vi "XYZ Control.vi"(1 "Wave Queue":refnum<queue>, 2 "Camera Queue":refnum<queue>, 3 "XYZ Controller":refnum<queue>) -> (0 "error out":errorcluster)   [LabVIEW 2016]
uses:
  controls/CameraControlTypeDef.ctl
  controls/Microscope Settings.ctl
  controls/ColourCalibration.ctl
  controls/ModeEnum.ctl
  controls/xy.ctl
  <vilib>/DAQmx/read.llb/DAQmx Read (Analog DBL 1Chan 1Samp).vi
  <vilib>/DAQmx/create/channels.llb/DAQmx Create Channel (AI-Voltage-Basic).vi
  <vilib>/DAQmx/miscellaneous.llb/DAQmx Fill In Error Info.vi
panel:
  in  "stop 2":bool
  in  "Z Position":dbl(slide) scale=-20000.0..20000.0 scale format="%#_6p"
  out "Z Position Read":dbl
  in  "End":dbl
  in  "Start":dbl
  in  "Step":dbl
  in  "Z Stack":bool
  in  "Delay /ms":dbl=100.0
  in  "Go to Current":bool
  in  "Clear List":bool
  in  "Add Current Position Highlighted":bool
  in  "Add Current Position":bool
  in  "Save Images":bool
  in  "Cycle Positions":bool
  in  "Coordinate List":i32(listbox)
  in  "Previous":bool
  in  "Next":bool
  out "Filter":i16
  out "Y Position Read":dbl
  out "X Position Read":dbl
  in  "Filter":dbl
  in  "Y Position":dbl(slide) scale=-20000.0..20000.0 scale format="%#_6p"
  in  "X Position":dbl(slide) scale=-20000.0..20000.0 scale format="%#_4p"
  in  "stop":bool
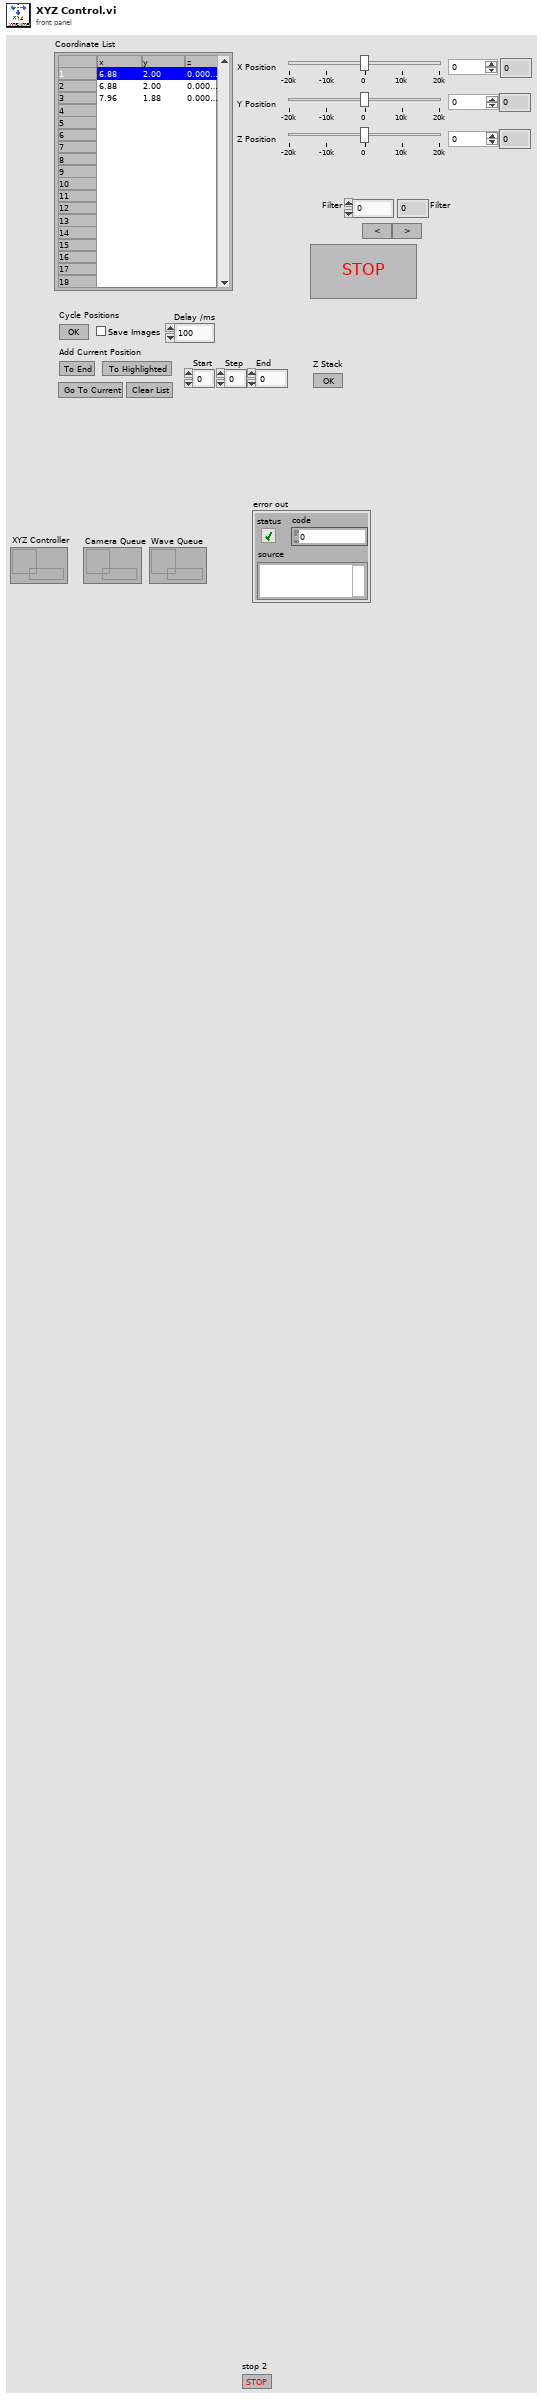
[diagram p1: front panel]
types:
  T1 = typedef "xy.ctl" = enum16{"Initalise", "setX", "getX", "setY", "getY", "stop", "setFilter", "getFilter", "FilterPrevious", "FilterNext", "setXYZ"}
  T2 = cluster{"State\n":T1, "X Position":dbl, "Y Position":dbl, "Filter":dbl, "Z Position":dbl}
  T3 = cluster{"Enum":T1, "X Position":dbl, "Y Position":dbl, "Filter":dbl, "Z Position":dbl}
  T4 = cluster{"State\n":T1, "X Position":dbl, "Y Position":dbl, dbl, "Filter":dbl}
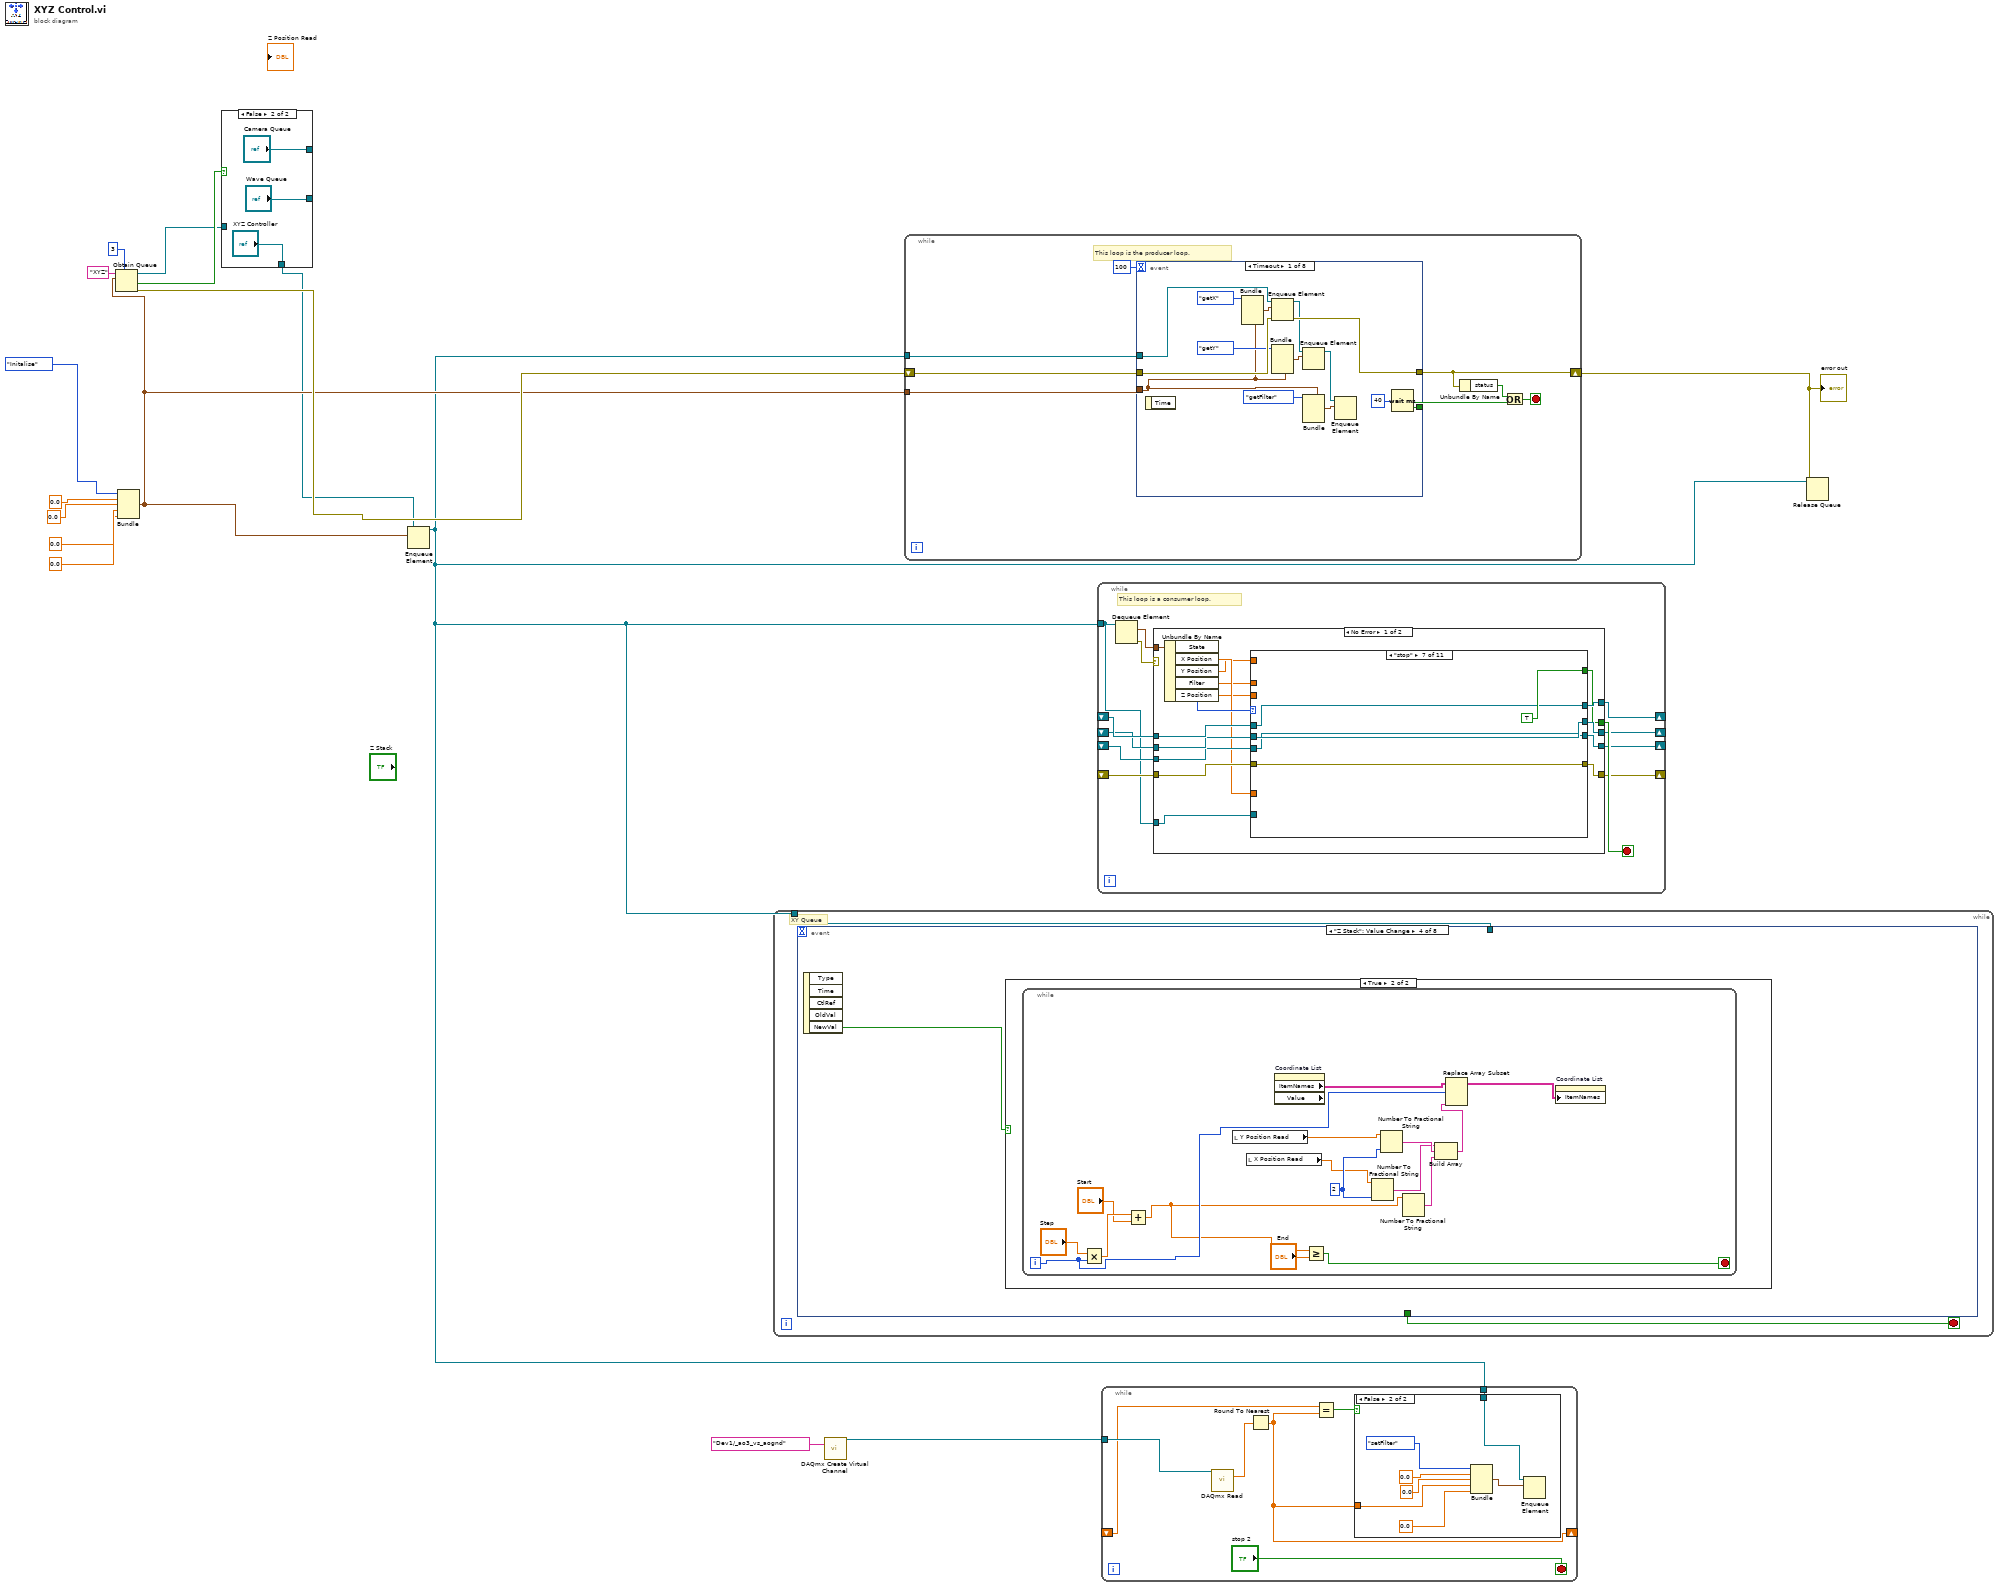
[diagram p0: block diagram]
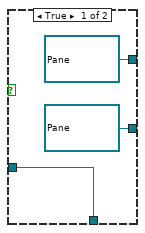
[diagram p3: hidden frame]
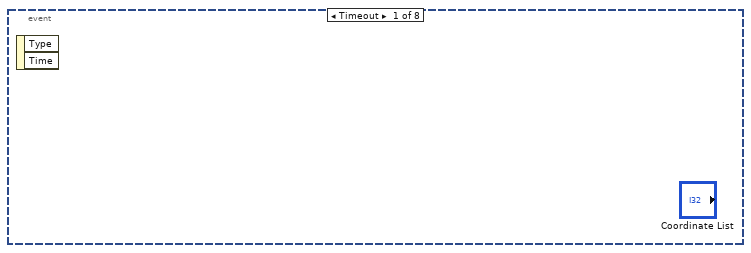
[diagram p4: hidden frame]
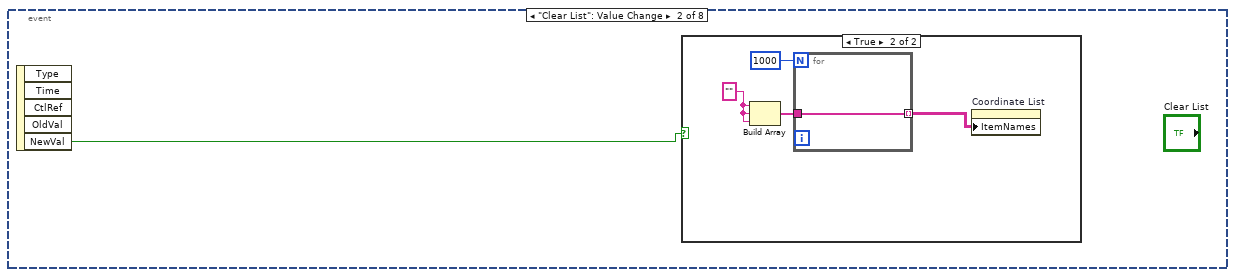
[diagram p5: hidden frame]
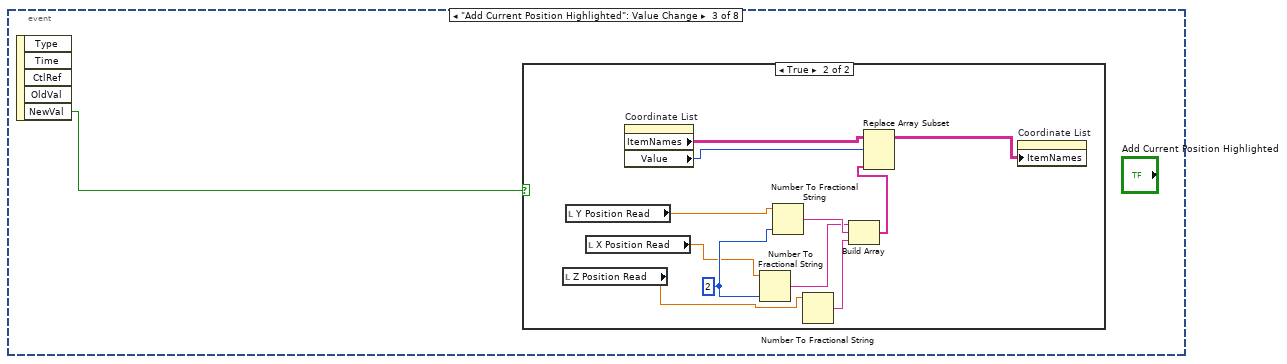
[diagram p7: hidden frame]
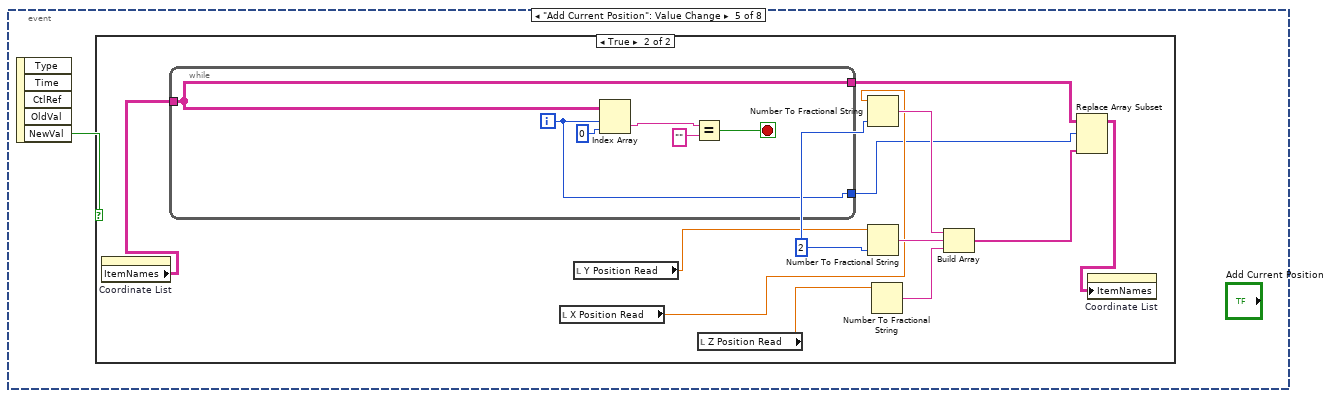
[diagram p10: hidden frame]
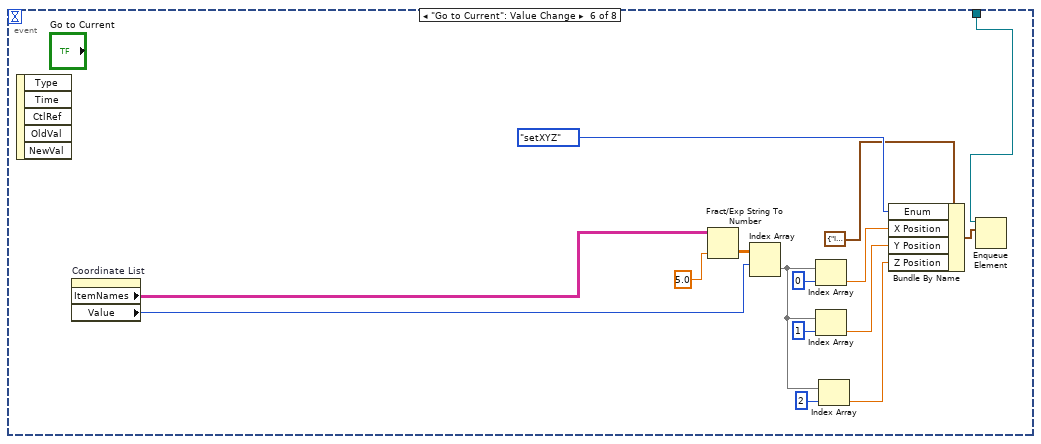
[diagram p12: hidden frame]
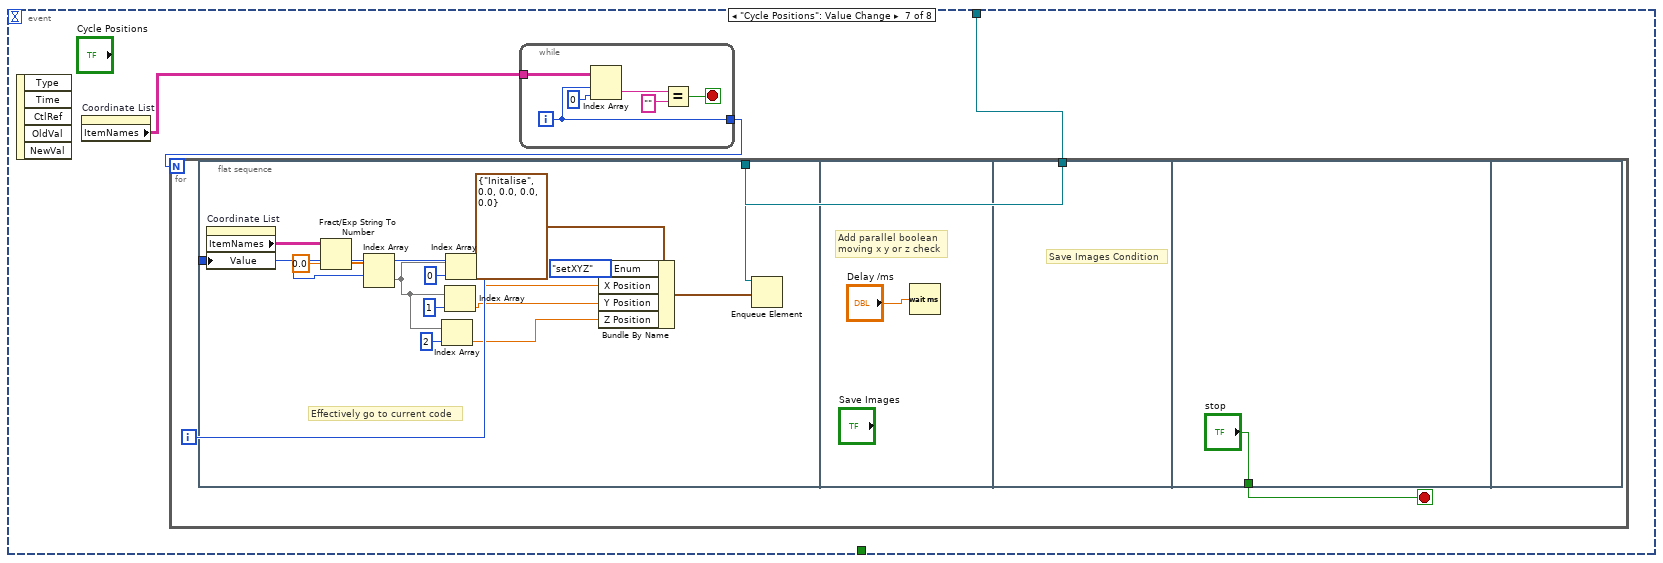
[diagram p13: hidden frame]
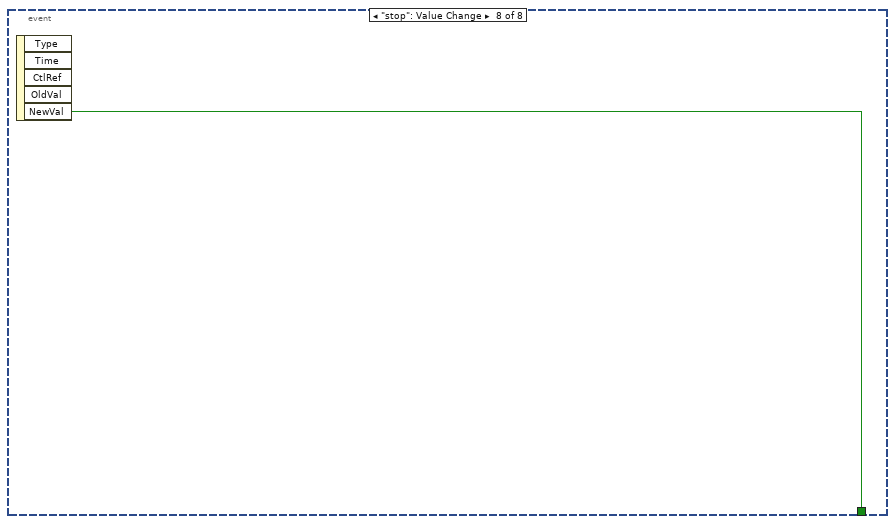
[diagram p14: hidden frame]
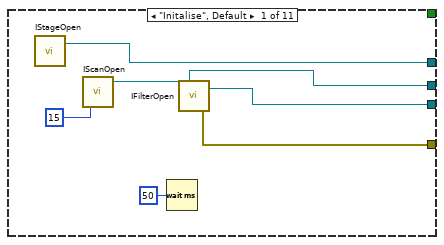
[diagram p15: hidden frame]
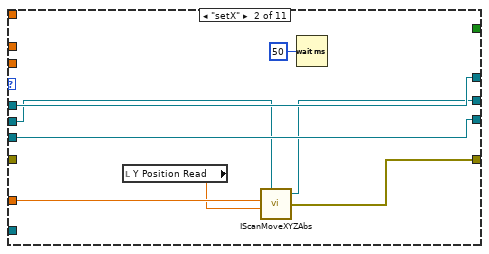
[diagram p16: hidden frame]
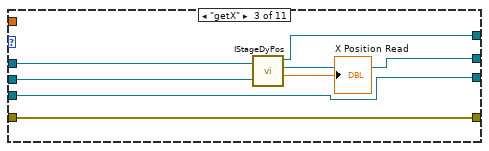
[diagram p17: hidden frame]
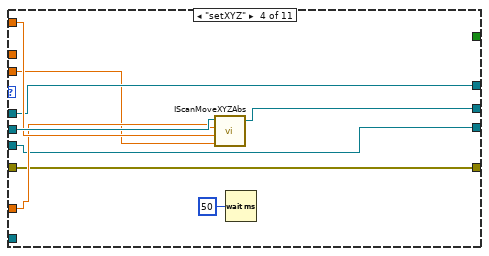
[diagram p18: hidden frame]
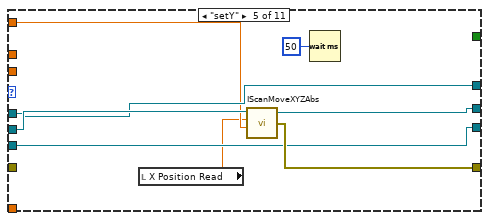
[diagram p19: hidden frame]
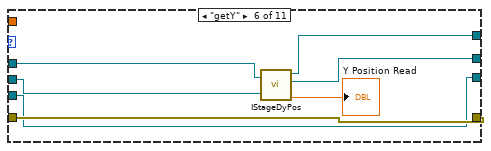
[diagram p20: hidden frame]
diagram:
  n1 = Bundle("State"=xy."Initalise", "X Position"=0.0, "Y Position"=0.0, "Filter"=0.0, "Z Position"=0.0) -> (w9:T2)  [unwired: 1 in]
  n2 = Obtain Queue(max queue size (-1, unlimited)=3, name (unnamed)="XYZ", element data type=w9) -> (queue out=w5:refnum<queue>, created new?=w6:bool, error out=w14:errorcluster)  [unwired: 2 in]
  n3 = case shown="False" w6 {
    tunnel: w5 -> [w19 _]
    tunnel: [w19 "XYZ Controller"] -> w4
    tunnel: [refnum<queue> refnum ("Wave Queue") "Wave Queue"] -> _
    tunnel: [refnum<queue> refnum ("Camera Queue") "Camera Queue"] -> _
    frame True {
    }
    frame False {
    }
  }
  n4 = Enqueue Element(queue=w4, element=w9) -> (queue out=w1:refnum<queue>)  [unwired: 2 in, 2 out]
  n5 = while {
    tunnel: w1 -> [w23]
    stop <- w24 stop-if-true
    # "XY Queue"
    n6 = event shown="[3] \"Z Stack\": Value Change" {
      selector: _ -> [_ _ _ _ _ _ _ _]
      dyn-events: _ -> [_ _ _ _ _ _ _ _]
      timeout: _ -> [_ _ _ _ _ _ _ _]
      tunnel: [_ _ _ _ _ _ _ w123] -> w24
      tunnel: w23 -> [_ _ _ _ _ w89 w94 _]
      event Timeout {
        n7 = event-data() -> ()  [unwired: 1 in, 2 out]
      }
      event "Clear List": Value Change {
        n8 = event-data() -> ("NewVal"=w25:bool)  [unwired: 1 in, 4 out]
        n9 = case shown="True" w25 {
          frame False {
          }
          frame True {
            w29 = "" ("y")
            n10 = Build Array(w29, w29, w29) -> (w27:string[])
            n11 = for {
              N: 1000 -> [_]
              tunnel: w27 -> [w30]
              tunnel: [w30] -> w26 mode=indexing
            }
            n12 = property on="Coordinate List" class="MCListbox (strict)"("ItemNames"=w26) -> ()  [unwired: 2 in, 2 out]
          }
        }
      }
      event "Add Current Position Highlighted": Value Change {
        n13 = event-data() -> ("NewVal"=w31:bool)  [unwired: 1 in, 4 out]
        n14 = case shown="True" w31 {
          frame False {
          }
          frame True {
            w39 = i16 2 ("width (-)")
            n15 = local read "Z Position Read"() -> (w32:dbl)
            n16 = local read "Y Position Read"() -> (w40:dbl)
            n17 = local read "X Position Read"() -> (w38:dbl)
            n18 = property on="Coordinate List" class="MCListbox (strict)"() -> ("ItemNames"=w41:string[][], "Value"=w42:i32)  [unwired: 2 in, 2 out]
            n19 = Number To Fractional String(number=w38, precision (6)=w39) -> (F-format string=w35:string)  [unwired: 2 in]
            n20 = Number To Fractional String(number=w40, precision (6)=w39) -> (F-format string=w36:string)  [unwired: 2 in]
            n21 = Number To Fractional String(number=w32) -> (F-format string=w37:string)  [unwired: 3 in]
            n22 = Build Array(w35, w36, w37) -> (w34:string[])
            n23 = Replace Array Subset(array=w41, new element=w34, index (row)=w42) -> (w33:string[][])  [unwired: 1 in]
            n24 = property on="Coordinate List" class="MCListbox (strict)"("ItemNames"=w33) -> ()  [unwired: 2 in, 2 out]
          }
        }
      }
      event "Z Stack": Value Change {
        n25 = event-data() -> ("NewVal"=w43:bool)  [unwired: 1 in, 4 out]
        n26 = case shown="True" w43 {
          frame False {
          }
          frame True {
            n27 = while {
              i -> [w58]
              stop <- w53 stop-if-true
              w50 = i16 2 ("width (-)")
              n28 = Multiply(x="Step", y=w58) -> (x*y=w57:dbl)
              n29 = Add(x=w57, y="Start") -> (x+y=w55:dbl)
              n30 = local read "Y Position Read"() -> (w51:dbl)
              n31 = local read "X Position Read"() -> (w49:dbl)
              n32 = property on="Coordinate List" class="MCListbox (strict)" props=["ItemNames", "Value"]() -> ("ItemNames"=w52:string[][])  [unwired: 2 in, 3 out]
              n33 = Greater Or Equal?(x=w55, y="End") -> (x >= y?=w53:bool)
              n34 = Number To Fractional String(number=w49, precision (6)=w50) -> (F-format string=w46:string)  [unwired: 2 in]
              n35 = Number To Fractional String(number=w51, precision (6)=w50) -> (F-format string=w47:string)  [unwired: 2 in]
              n36 = Number To Fractional String(number=w55) -> (F-format string=w48:string)  [unwired: 3 in]
              n37 = Build Array(w46, w47, w48) -> (w45:string[])
              n38 = Replace Array Subset(array=w52, new element=w45, index (row)=w58) -> (w44:string[][])  [unwired: 1 in]
              n39 = property on="Coordinate List" class="MCListbox (strict)"("ItemNames"=w44) -> ()  [unwired: 2 in, 2 out]
            }
          }
        }
      }
      event "Add Current Position": Value Change {
        n40 = event-data() -> ("NewVal"=w60:bool)  [unwired: 1 in, 4 out]
        n41 = case shown="True" w60 {
          frame False {
          }
          frame True {
            w69 = i16 2 ("precision (6)")
            n42 = property on="Coordinate List" class="MCListbox (strict)"() -> ("ItemNames"=w66:string[][])  [unwired: 2 in, 2 out]
            n43 = while {
              tunnel: [w75] -> w63
              tunnel: w66 -> [w74]
              tunnel: [w74] -> w65
              i -> [w75]
              stop <- w76 stop-if-true
              n44 = Index Array(array=w74, index (row)=w75, index (col)=0 ("disabled index (col)")) -> (element=w73:string)
              n45 = Equal?(x=w73, y="") -> (x = y?=w76:bool)
            }
            n46 = local read "X Position Read"() -> (w68:dbl)
            n47 = local read "Y Position Read"() -> (w67:dbl)
            n48 = local read "Z Position Read"() -> (w61:dbl)
            n49 = Number To Fractional String(number=w68, precision (6)=w69) -> (F-format string=w72:string)  [unwired: 2 in]
            n50 = Number To Fractional String(number=w67, precision (6)=w69) -> (F-format string=w70:string)  [unwired: 2 in]
            n51 = Number To Fractional String(number=w61) -> (F-format string=w71:string)  [unwired: 3 in]
            n52 = Build Array(w72, w70, w71) -> (w64:string[])
            n53 = Replace Array Subset(array=w65, new element=w64, index (row)=w63) -> (w62:string[][])  [unwired: 1 in]
            n54 = property on="Coordinate List" class="MCListbox (strict)"("ItemNames"=w62) -> ()  [unwired: 2 in, 2 out]
          }
        }
      }
      event "Go to Current": Value Change {
        n55 = event-data() -> ()  [unwired: 1 in, 5 out]
        n56 = property on="Coordinate List" class="MCListbox (strict)"() -> ("ItemNames"=w93:string[][], "Value"=w82:i32)  [unwired: 2 in, 2 out]
        n57 = Fract/Exp String To Number(string=w93, default (0 dbl)=5.0 ("default (0 DBL)")) -> (number=w92:dbl[][])  [unwired: 2 in, 1 out]
        n58 = Index Array(array=w92, index (row)=w82) -> (element=w80:dbl[])  [unwired: 1 in]
        n59 = Index Array(array=w80, index=0) -> (element=w84:dbl)
        n60 = Index Array(array=w80, index=1) -> (element=w85:dbl)
        n61 = Index Array(array=w80, index=2) -> (element=w79:dbl)
        n62 = Bundle By Name(cluster=T3 {"Enum"=enum."Initalise", "X Position"=0.0, "Y Position"=0.0, "Filter"=0.0, "Z Position"=0.0} ("element"), "Enum"=xy."setXYZ", "X Position"=w84, "Y Position"=w85, "Z Position"=w79) -> (w86:T3)
        n63 = Enqueue Element(queue=w89, element=w86) -> ()  [unwired: 2 in, 3 out]
      }
      event "Cycle Positions": Value Change {
        n64 = event-data() -> ()  [unwired: 1 in, 5 out]
        n65 = property on="Coordinate List" class="MCListbox (strict)"() -> ("ItemNames"=w96:string[][])  [unwired: 2 in, 2 out]
        n66 = while {
          tunnel: w96 -> [w122]
          tunnel: [w117] -> w95
          i -> [w117]
          stop <- w118 stop-if-true
          n67 = Index Array(array=w122, index (row)=w117, index (col)=0 ("disabled index (col)")) -> (element=w120:string)
          n68 = Equal?(x=w120, y="") -> (x = y?=w118:bool)
        }
        n69 = for {
          N: w95 -> [_]
          tunnel: w94 -> [w99]
          i -> [w98]
          stop <- w97 stop-if-true
          n70 = flat-sequence {
            tunnel: w99 -> [w103]
            tunnel: w98 -> [w101]
            tunnel: ["stop"] -> w97
            frame #0 {
              # "Effectively go to current code"
              n71 = property on="Coordinate List" class="MCListbox (strict)"("Value"=w101) -> ("ItemNames"=w102:string[][])  [unwired: 2 in, 2 out]
              n72 = Fract/Exp String To Number(string=w102, default (0 dbl)=0.0 ("default (0 DBL)")) -> (number=w114:dbl[][])  [unwired: 2 in, 1 out]
              n73 = Index Array(array=w114, index (row)=w101) -> (element=w112:dbl[])  [unwired: 1 in]
              n74 = Index Array(array=w112, index=2) -> (element=w100:dbl)
              n75 = Index Array(array=w112, index=1) -> (element=w106:dbl)
              n76 = Index Array(array=w112, index=0) -> (element=w107:dbl)
              n77 = Bundle By Name(cluster=T3 {"Enum"=enum."Initalise", "X Position"=0.0, "Y Position"=0.0, "Filter"=0.0, "Z Position"=0.0} ("element"), "Enum"=xy."setXYZ", "X Position"=w107, "Y Position"=w106, "Z Position"=w100) -> (w104:T3)
              n78 = Enqueue Element(queue=w103, element=w104) -> ()  [unwired: 2 in, 3 out]
            }
            frame #1 {
              # "Add parallel boolean\nmoving x y or z check"
              n79 = Wait (ms)(milliseconds to wait="Delay /ms") -> ()  [unwired: 1 out]
            }
            frame #2 {
              # "Save Images Condition"
            }
            frame #3 {
            }
            frame #4 {
            }
          }
        }
      }
      event "stop": Value Change {
        n80 = event-data() -> ("NewVal"=w123:bool)  [unwired: 1 in, 4 out]
      }
    }
  }
  n81 = call-poly <vilib>:"DAQmx Create Virtual Channel.vi"("physical channels"=tag "Dev1/_ao3_vs_aognd") -> ("task out"=w3:refnum<k21>)  [unwired: 13 in, 1 out]
  n82 = while {
    shift-right: [w127] -> w16
    shift-left: w14 -> [w130]
    tunnel: w1 -> [w131]
    tunnel: w9 -> [w125]
    stop <- w128 stop-if-true
    # "This loop is the producer loop."
    n83 = event shown="[0] Timeout" {
      selector: _ -> [_ _ _ _ _ _ _ _]
      dyn-events: _ -> [_ _ _ _ _ _ _ _]
      timeout: 100 -> [_ _ _ _ _ _ _ _]
      tunnel: w131 -> [w144 w148 w154 w163 w170 w173 w180 w191]
      tunnel: w130 -> [w143 w145 w153 w159 w169 _ _ w190]
      tunnel: [w140 _ _ w158 w167 _ _ w187] -> w127
      tunnel: [_ _ _ TRUE ("stop") _ _ _ _] -> w129
      tunnel: w125 -> [w139 w146 w152 w162 w168 w172 w179 w189]
      event Timeout {
        n84 = event-data() -> ()  [unwired: 1 in, 1 out]
        n85 = Bundle(cluster=w139, "State"=xy."getX") -> (w136:T2)  [unwired: 4 in]
        n86 = Enqueue Element(queue=w144, element=w136, error in (no error)=w143) -> (queue out=w137:refnum<queue>, error out=w140:errorcluster)  [unwired: 1 in, 1 out]
        n87 = Bundle(cluster=w139, "State"=xy."getY") -> (w135:T2)  [unwired: 4 in]
        n88 = Enqueue Element(queue=w137, element=w135) -> (queue out=w134:refnum<queue>)  [unwired: 2 in, 2 out]
        n89 = Bundle(cluster=w139, "State"=xy."getFilter") -> (w133:T2)  [unwired: 4 in]
        n90 = Enqueue Element(queue=w134, element=w133) -> ()  [unwired: 2 in, 3 out]
        n91 = Wait (ms)(milliseconds to wait=u32 40) -> ()  [unwired: 1 out]
      }
      event "Z Position": Value Change {
        n92 = event-data() -> ()  [unwired: 1 in, 2 out]
        n93 = Bundle(cluster=w146, "State"=xy."setX", "X Position"="Z Position") -> (w149:T2)  [unwired: 3 in]
        n94 = Enqueue Element(queue=w148, element=w149, error in (no error)=w145) -> ()  [unwired: 1 in, 3 out]
      }
      event "X Position": Value Change {
        n95 = event-data() -> ()  [unwired: 1 in, 1 out]
        n96 = Bundle(cluster=w152, "State"=xy."setX", "X Position"="X Position") -> (w155:T2)  [unwired: 3 in]
        n97 = Enqueue Element(queue=w154, element=w155, error in (no error)=w153) -> ()  [unwired: 1 in, 3 out]
      }
      event "stop": Value Change {
        n98 = event-data() -> ()  [unwired: 1 in, 1 out]
        n99 = Bundle(cluster=w162, "State"=xy."stop") -> (w160:T2)  [unwired: 4 in]
        n100 = Enqueue Element At Opposite End(queue=w163, element=w160, error in (no error)=w159) -> (error out=w158:errorcluster)  [unwired: 1 in, 2 out]
      }
      event "Filter": Value Change {
        n101 = event-data() -> ()  [unwired: 1 in, 1 out]
        n102 = Bundle(cluster=w168, "State"=xy."setFilter", "Filter"="Filter") -> (w166:T2)  [unwired: 3 in]
        n103 = Enqueue Element(queue=w170, element=w166, error in (no error)=w169) -> (error out=w167:errorcluster)  [unwired: 1 in, 2 out]
      }
      event "Next": Value Change {
        n104 = event-data() -> ()  [unwired: 1 in, 1 out]
        n105 = case shown="True" "Next" {
          tunnel: w173 -> [_ w176]
          tunnel: w172 -> [_ w175]
          frame False {
          }
          frame True {
            n106 = Bundle(cluster=w175, "State"=xy."FilterNext") -> (w174:T2)  [unwired: 4 in]
            n107 = Enqueue Element(queue=w176, element=w174) -> ()  [unwired: 2 in, 3 out]
          }
        }
      }
      event "Previous": Value Change {
        n108 = event-data() -> ()  [unwired: 1 in, 1 out]
        n109 = case shown="True" "Previous" {
          tunnel: w180 -> [_ w183]
          tunnel: w179 -> [_ w182]
          frame False {
          }
          frame True {
            n110 = Bundle(cluster=w182, "State"=xy."FilterPrevious") -> (w181:T2)  [unwired: 4 in]
            n111 = Enqueue Element(queue=w183, element=w181) -> ()  [unwired: 2 in, 3 out]
          }
        }
      }
      event "Y Position": Value Change {
        n112 = event-data() -> ()  [unwired: 1 in, 1 out]
        n113 = Bundle(cluster=w189, "State"=xy."setY", "Y Position"="Y Position") -> (w188:T2)  [unwired: 3 in]
        n114 = Enqueue Element(queue=w191, element=w188, error in (no error)=w190) -> (error out=w187:errorcluster)  [unwired: 1 in, 2 out]
      }
    }
    n115 = Unbundle By Name(w127) -> ("status"=w126:bool)
    n116 = Or(x=w126, y=w129) -> (x .or. y?=w128:bool)
  }
  "error out" <- w16
  n117 = while {
    tunnel: w1 -> [w192]
    shift-right: [w200] -> _
    shift-left: _ -> [w197]
    shift-right: [w199] -> _
    shift-left: _ -> [w196]
    shift-right: [w198] -> _
    shift-left: _ -> [w195]
    shift-right: [w194] -> _
    shift-left: _ -> [w193]
    stop <- w201 stop-if-true
    # "This loop is a consumer loop."
    n118 = Dequeue Element(queue=w192) -> (element=w202:T2, error out=w203:errorcluster)  [unwired: 2 in, 2 out]
    n119 = case shown="No Error" w203 {
      tunnel: w202 -> [w219 _]
      tunnel: [w209 TRUE] -> w201
      tunnel: [w217 _] -> w200
      tunnel: [w216 _] -> w199
      tunnel: [w215 _] -> w198
      tunnel: w197 -> [w214 _]
      tunnel: w196 -> [w213 _]
      tunnel: w195 -> [w212 _]
      tunnel: [w211 w294] -> w194
      tunnel: w193 -> [w210 w294]
      tunnel: w192 -> [w206 _]
      frame No Error {
        n120 = Unbundle By Name(w219) -> ("State"=w218:T1, "X Position"=w208:dbl, "Y Position"=w207:dbl, "Filter"=w204:dbl, "Z Position"=w205:dbl)
        n121 = case shown="\"stop\"" w218 {
          tunnel: [w225 w233 w238 w245 w254 w262 w267 w271 w277 w286 w289] -> w217
          tunnel: [w224 w229 w237 w246 w256 w261 w266 w272 w278 w287 w288] -> w216
          tunnel: [w223 w232 w235 w244 w253 w259 w265 w275 w279 w283 w292] -> w215
          tunnel: w214 -> [_ w233 w240 w245 w254 w264 w267 w271 w277 w286 w289]
          tunnel: w213 -> [_ w230 w239 w249 w257 w263 w266 w272 w278 w287 w288]
          tunnel: w212 -> [_ w232 w235 w244 w253 w259 w265 w274 w280 w284 w293]
          tunnel: [w222 w228 w236 w243 w255 w260 w269 w270 w281 w282 w291] -> w211
          tunnel: w210 -> [_ _ w236 w243 _ w260 w269 _ _ _ _]
          tunnel: [_ _ _ _ _ _ TRUE _ _ _ _] -> w209
          tunnel: w208 -> [_ w231 _ w247 _ _ _ _ _ _ _]
          tunnel: w207 -> [_ _ _ w248 w252 _ _ _ _ _ _]
          tunnel: w206 -> [_ _ _ _ _ _ _ _ _ _ _]
          tunnel: w205 -> [_ _ _ w241 _ _ _ _ _ _ _]
          tunnel: w204 -> [_ _ _ _ _ _ _ _ _ _ w290]
          frame "Initalise", Default {
            n122 = call "IStageOpen.vi"() -> ("PRIORLib.IStageOut"=w225:refnum<k7>)  [unwired: 1 in, 1 out]
            n123 = call "IScanOpen.vi"("Port"=15) -> ("PRIORLib.IScanOut"=w224:refnum<k7>)  [unwired: 2 out]
            n124 = Wait (ms)(milliseconds to wait=u32 50) -> ()  [unwired: 1 out]
            n125 = call "IFilterOpen.vi"() -> ("PRIORLib.IFilterOut"=w223:refnum<k7>, "error out"=w222:errorcluster)  [unwired: 1 in]
          }
          frame "setX" {
            n126 = local read "Y Position Read"() -> (w227:dbl)
            n127 = call "IScanMoveXYZAbs.vi"("YPos"=w227, "XPos"=w231, "PRIORLib.IScanIn"=w230) -> ("error out"=w228:errorcluster, "PRIORLib.IScanOut"=w229:refnum<k7>)  [unwired: 1 in, 1 out]
            n128 = Wait (ms)(milliseconds to wait=u32 50) -> ()  [unwired: 1 out]
          }
          frame "getX" {
            n129 = call "IStageDyPos.vi"("PRIORLib.IStageIn"=w240, "PRIORLib.IScanIn"=w239) -> ("PRIORLib.IStageOut"=w238:refnum<k7>, "PRIORLib.IScanOut"=w237:refnum<k7>, "XPos"=→"X Position Read":dbl)  [unwired: 1 out]
          }
          frame "setXYZ" {
            n130 = call "IScanMoveXYZAbs.vi"("ZPos"=w241, "YPos"=w248, "XPos"=w247, "PRIORLib.IScanIn"=w249) -> ("PRIORLib.IScanOut"=w246:refnum<k7>)  [unwired: 2 out]
            n131 = Wait (ms)(milliseconds to wait=u32 50) -> ()  [unwired: 1 out]
          }
          frame "setY" {
            n132 = local read "X Position Read"() -> (w251:dbl)
            n133 = call "IScanMoveXYZAbs.vi"("YPos"=w252, "XPos"=w251, "PRIORLib.IScanIn"=w257) -> ("error out"=w255:errorcluster, "PRIORLib.IScanOut"=w256:refnum<k7>)  [unwired: 1 in, 1 out]
            n134 = Wait (ms)(milliseconds to wait=u32 50) -> ()  [unwired: 1 out]
          }
          frame "getY" {
            n135 = call "IStageDyPos.vi"("PRIORLib.IStageIn"=w264, "PRIORLib.IScanIn"=w263) -> ("PRIORLib.IStageOut"=w262:refnum<k7>, "PRIORLib.IScanOut"=w261:refnum<k7>, "YPos"=→"Y Position Read":dbl)  [unwired: 1 out]
          }
          frame "stop" {
          }
          frame "getFilter" {
            n136 = call "IFilterPosition.vi"("PRIORLib.IFilterIn"=w274) -> ("PRIORLib.IFilterOut"=w275:refnum<k7>, "error out"=w270:errorcluster, "Position"=→"Filter":i16)  [unwired: 1 in]
          }
          frame "FilterPrevious" {
            n137 = Wait (ms)(milliseconds to wait=u32 50) -> ()  [unwired: 1 out]
            n138 = call "IFilterPrevious.vi"("PRIORLib.IFilterIn"=w280) -> ("PRIORLib.IFilterrOut"=w279:refnum<k7>, "error out"=w281:errorcluster)  [unwired: 1 in, 1 out]
          }
          frame "FilterNext" {
            n139 = call "IFilterNext.vi"("PRIORLib.IFilterIn"=w284) -> ("PRIORLib.IFilterrOut"=w283:refnum<k7>, "error out"=w282:errorcluster)  [unwired: 1 in, 1 out]
            n140 = Wait (ms)(milliseconds to wait=u32 50) -> ()  [unwired: 1 out]
          }
          frame "setFilter" {
            n141 = call "IFilterPut.vi"("PRIORLib.IFilterIn"=w293, "Position"=w290) -> ("PRIORLib.IFilterrOut"=w292:refnum<k7>, "error out"=w291:errorcluster)  [unwired: 1 out]
          }
        }
      }
      frame Error {
        # "Return true in any case that should stop the loop."
      }
    }
  }
  n142 = while {
    tunnel: w3 -> [w302]
    shift-right: [w297] -> _
    shift-left: _ -> [w299]
    tunnel: w1 -> [w296]
    stop <- "stop 2" stop-if-true
    n143 = call-poly <vilib>:"DAQmx Read.vi"("task/channels in"=w302) -> ("data"=w300:dbl)  [unwired: 12 in, 2 out]
    n144 = Round To Nearest(number=w300) -> (nearest integer value=w297:dbl)
    n145 = Equal?(x=w299, y=w297) -> (x = y?=w298:bool)
    n146 = case shown="False" w298 {
      tunnel: w297 -> [_ w303]
      tunnel: w296 -> [_ w305]
      frame True {
      }
      frame False {
        n147 = Bundle("State"=xy."setFilter", "X Position"=0.0, "Y Position"=0.0, w303, "Filter"=0.0) -> (w306:T4)  [unwired: 1 in]
        n148 = Enqueue Element(queue=w305, element=w306) -> ()  [unwired: 2 in, 3 out]
      }
    }
  }
  n149 = Release Queue(queue=w1, error in (no error)=w16) -> ()  [unwired: 1 in, 3 out]
